vi "Load Test Tag from File.vi"(6 "AllTests":refnum<class>[](array[class]), 7 "Tree reference":refnum<vi>, 8 "error in":errorcluster, 9 "TestTag":string) -> (0 "error out":errorcluster, 1 "Test Tag Test":refnum<class>)   [LabVIEW 2011, in "GraphicalTestRunner.lvlib"]
uses:
  GraphicalTestRunner.lvlib
  Classes/TestSuite/TestSuite.lvclass
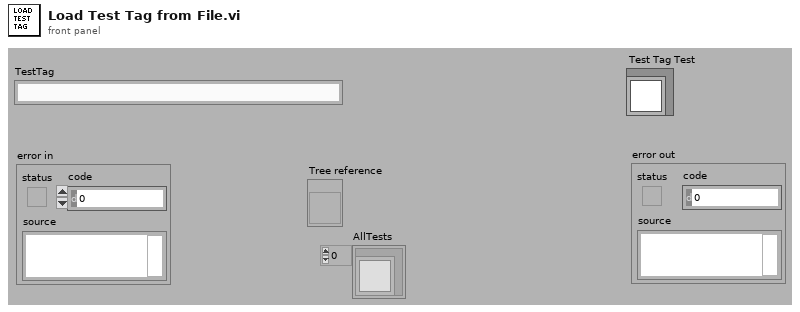
[diagram p1: front panel]
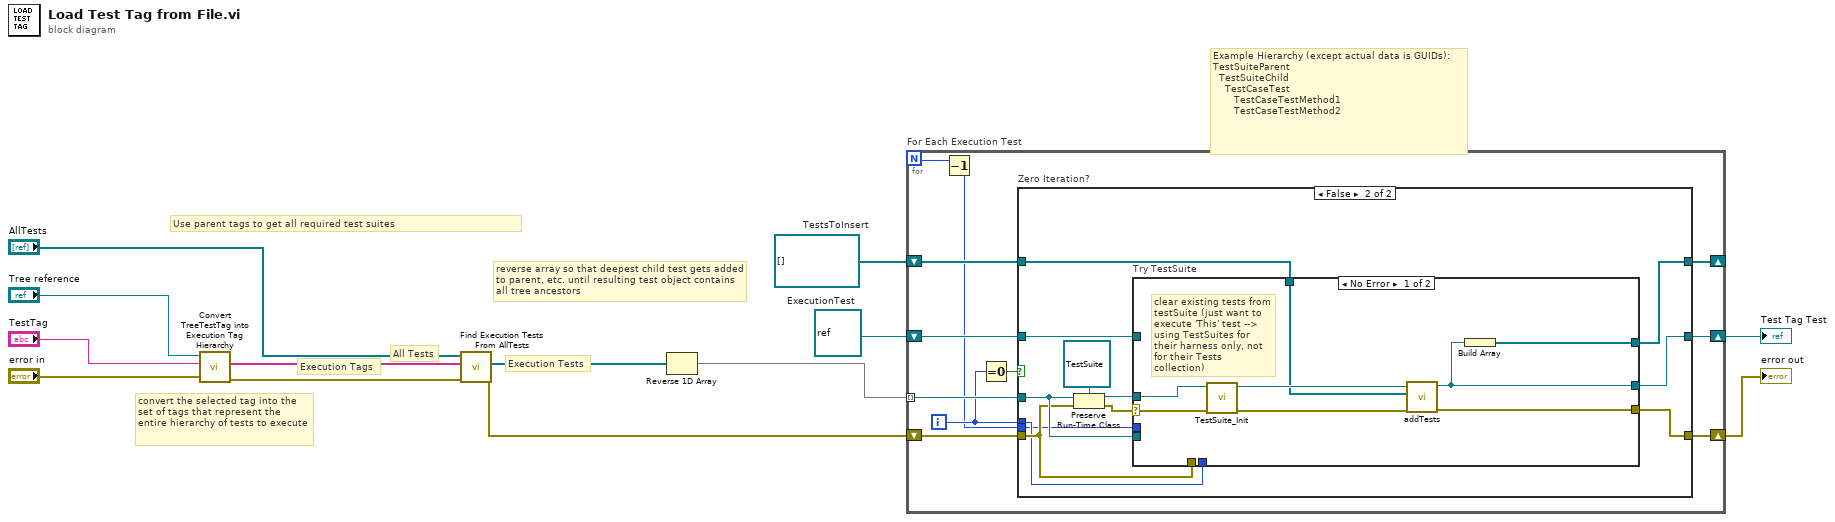
[diagram p0: block diagram]
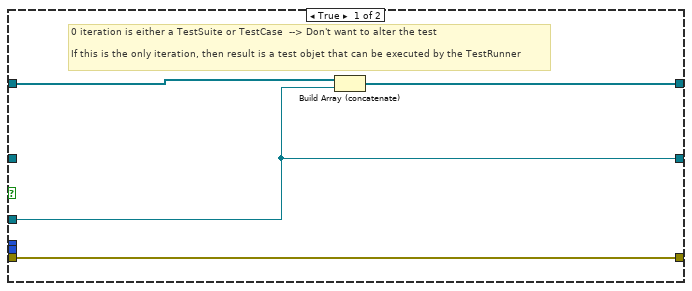
[diagram p2: hidden frame]
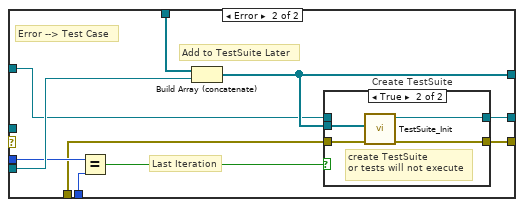
[diagram p3: hidden frame]
diagram:
  w2 = refnum<class>[] []  # TestsToInsert
  w1 = refnum<class> refnum  # ExecutionTest
  # "reverse array so that deepest child test gets added to parent, etc. until resulting test object contains all tree ancestors"
  # "Execution Tests"
  # "All Tests"
  # "Execution Tags"
  # "convert the selected tag into the set of tags that represent the entire hierarchy of tests to execute"
  # "Example Hierarchy (except actual data is GUIDs):\nTestSuiteParent\n  TestSuiteChild\n    TestCaseTest\n       TestCaseTestMethod1\n       TestCaseTestMethod2"
  # "Use parent tags to get all required test suites"
  n1 = call "Convert TreeTestTag into Execution Tag Hierarchy.vi"("error in"="error in", "TestTag"="TestTag", "Tree reference"="Tree reference") -> ("error out"=w6:errorcluster, "Test Tags to Execute"=w8:string[])  [unwired: 7 in]
  n2 = call "Find Execution Tests From AllTests.vi"("error in"=w6, "Test Tags to Execute"=w8, "AllTests"="AllTests") -> ("error out"=w5:errorcluster, "ExecutionTests"=w9:refnum<class>[])  [unwired: 7 in]
  n3 = Reverse 1D Array(array=w9) -> (reversed array=w4:refnum<class>[])
  n4 = for "For Each Execution Test" {
    N -> [w15]
    tunnel: w4 -> [w24] mode=indexing
    shift-right: [w23] -> w3
    shift-left: w1 -> [w18]
    shift-right: [w20] -> w7
    shift-left: w5 -> [w19]
    shift-right: [w16] -> _
    shift-left: w2 -> [w17]
    i -> [w22]
    n5 = Decrement(x=w15) -> (x-1=w14:i32)
    n6 = Equal To 0?(x=w22) -> (x = 0?=w21:bool)
    n7 = case "Zero Iteration?" shown="False" w21 {
      tunnel: w24 -> [w25 w33]
      tunnel: [w25 w35] -> w23
      tunnel: w22 -> [_ w30]
      tunnel: [w27 w36] -> w20
      tunnel: w19 -> [w27 w31]
      tunnel: w18 -> [_ w32]
      tunnel: w17 -> [w28 w37]
      tunnel: [w26 w34] -> w16
      tunnel: w14 -> [_ w29]
      frame True {
        # "0 iteration is either a TestSuite or TestCase  --> Don't want to alter the test\n\nIf this is the only iteration, then result is a test objet that can be executed by the TestRunner"
        n8 = Build Array (concatenate)(w28, w25) -> (w26:refnum<class>[])
      }
      frame False {
        n9 = Preserve Run-Time Class(object in=w33, error in=w31, 2:refnum<class "TestSuite.lvclass"> refnum ("TestSuite in")) -> (object out=w39:refnum<class "TestSuite.lvclass">, error out=w38:errorcluster)
        n10 = case "Try TestSuite" shown="No Error" w38 {
          selector: w38 -> [w41 _]
          tunnel: w39 -> [w48 _]
          tunnel: w37 -> [w46 w58]
          tunnel: [w44 w49] -> w36
          tunnel: [w43 w52] -> w35
          tunnel: [w42 w53] -> w34
          tunnel: w33 -> [_ w57]
          tunnel: w32 -> [_ w51]
          tunnel: w31 -> [_ w50]
          tunnel: w30 -> [_ w56]
          tunnel: w29 -> [_ w55]
          frame No Error {
            # "clear existing tests from testSuite (just want to execute 'This' test --> using TestSuites for their harness only, not for their Tests collection)"
            n11 = call "TestSuite_Init.vi"("error in (no error)"=w41, "TestSuite in"=w48) -> ("error out"=w45:errorcluster, "TestSuite out"=w47:refnum<class "TestSuite.lvclass">)  [unwired: 8 in]
            n12 = call-dynamic "addTests.vi"("error in (no error)"=w45, "tests"=w46, "TestSuite in"=w47) -> ("error out"=w44:errorcluster, "TestSuite out"=w43:refnum<class "TestSuite.lvclass">)  [unwired: 7 in]
            n13 = Build Array(w43) -> (w42:refnum<class "TestSuite.lvclass">[])
          }
          frame Error {
            # "Last Iteration"
            # "Add to TestSuite Later"
            # "Error --> Test Case"
            n14 = Equal?(x=w55, y=w56) -> (x = y?=w54:bool)
            n15 = Build Array (concatenate)(w58, w57) -> (w53:refnum<class>[])
            n16 = case "Create TestSuite" shown="True" w54 {
              tunnel: w53 -> [_ w64]
              tunnel: [w60 w63] -> w52
              tunnel: w51 -> [w60 _]
              tunnel: w50 -> [w59 w62]
              tunnel: [w59 w61] -> w49
              frame False {
              }
              frame True {
                # "create TestSuite\nor tests will not execute"
                n17 = call "TestSuite_Init.vi"("error in (no error)"=w62, "tests (none)"=w64) -> ("error out"=w61:errorcluster, "TestSuite out"=w63:refnum<class "TestSuite.lvclass">)  [unwired: 8 in]
              }
            }
          }
        }
      }
    }
  }
  "Test Tag Test" <- w3
  "error out" <- w7
